vi "BinaryOutput.vi"(8 "Current Threshold":dbl=1000.0 format="%#_13g") -> (2 "Actual Binary\nOutput":bool[](array[boolean]), 11 "Current Level of Output Pins":dbl[](array[numeric]))   [LabVIEW 2018]
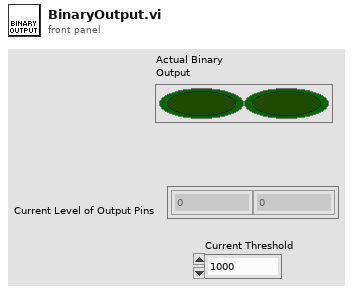
[diagram p1: front panel]
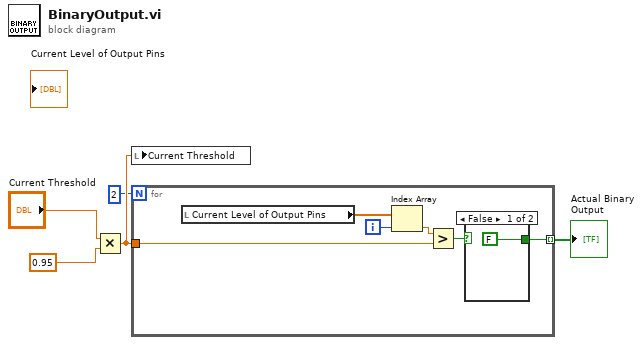
[diagram p0: block diagram]
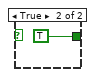
[diagram p2: hidden frame]
diagram:
  n1 = Multiply(x="Current Threshold", y=0.95) -> (x*y=w2:dbl)
  n2 = local write "Current Threshold"(w2) -> ()
  n3 = for {
    N: 2 -> [_]
    tunnel: w2 -> [w8]
    tunnel: [w6] -> w5 mode=indexing
    i -> [w7]
    n4 = local read "Current Level of Output Pins"() -> (w10:dbl[])
    n5 = Index Array(array=w10, index=w7) -> (element=w9:dbl)
    n6 = Greater?(x=w9, y=w8) -> (0:w11:bool)
    n7 = case shown="False" w11 {
      tunnel: [FALSE TRUE] -> w6
      frame False {
      }
      frame True {
      }
    }
  }
  "Actual Binary\nOutput" <- w5
